vi "Set Video Mode.vi"(6 "Flags":u32, 8 "error in":errorcluster, 9 "BPP":i32=8, 10 "Height":i32=480, 11 "Width":i32=640) -> (0 "error out":errorcluster, 3 "Screen Pointer":u32)   [LabVIEW 2014, in "LibSDL2.lvlib"]
uses:
  LibSDL2.lvlib
  DLL/SDL2.dll
panel:
  out "value":i32
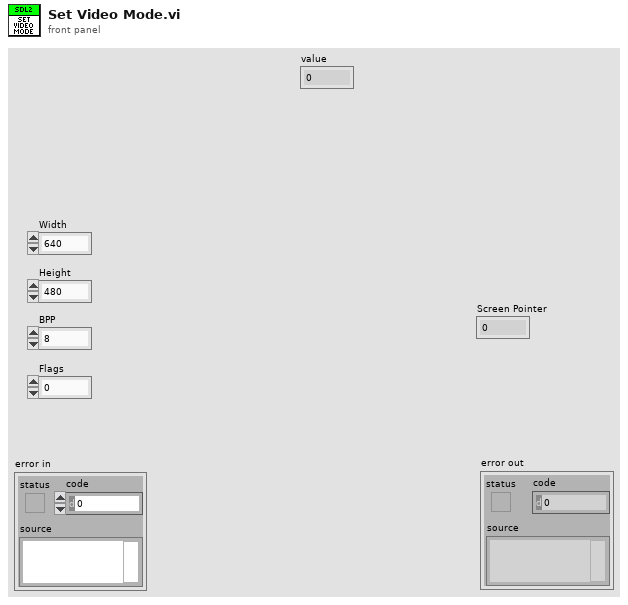
[diagram p1: front panel]
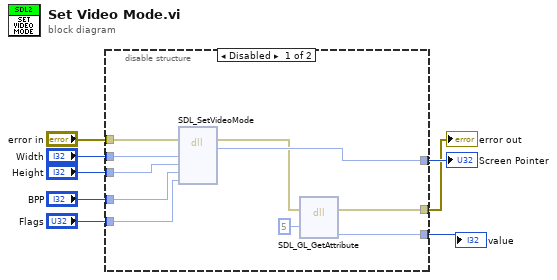
[diagram p0: block diagram]
diagram:
  n1 = disable-structure shown="Disabled" {
    disable-tunnel: "Flags" -> [w18 _]
    disable-tunnel: "BPP" -> [w17 _]
    disable-tunnel: "Height" -> [w16 _]
    disable-tunnel: "Width" -> [w15 _]
    disable-tunnel: "error in" -> [w14 _]
    disable-tunnel: [w13 _] -> w3
    disable-tunnel: [w11 _] -> w2
    disable-tunnel: [w9 _] -> w1
    frame Disabled {
      n2 = dll-call lib="C:/dev/PGS/LabSDL2/Source/LibSDL2 Wrapper/DLL/SDL2.dll" fn="SDL_SetVideoMode"(error in=w14, "width"=w15, "height"=w16, "bpp"=w17, "flags"=w18) -> (error out=w12:errorcluster, "return type"=w13:u32)  [unwired: 6 in, 1 out]
      n3 = dll-call lib="C:/dev/PGS/LabSDL2/Source/LibSDL2 Wrapper/DLL/SDL2.dll" fn="SDL_GL_GetAttribute"(error in=w12, "attribute"=u32 5) -> (error out=w11:errorcluster, "value"=w9:i32)  [unwired: 5 in, 1 out]
    }
    frame Enabled {
    }
  }
  "error out" <- w2
  "Screen Pointer" <- w3
  "value" <- w1
